vi "cumplimiento.vi"(8 "error in (no error)":errorcluster, 11 "Prueba07 in":refnum<class "Prueba07.lvclass">) -> (0 "error out":errorcluster, 3 "Prueba07 out":refnum<class "Prueba07.lvclass">)   [LabVIEW 2019, in "Prueba07.lvclass"]
uses:
  Prueba07.lvclass
  Prueba07.lvclass/Prueba07.ctl
panel:
  out "cumpimiento":string
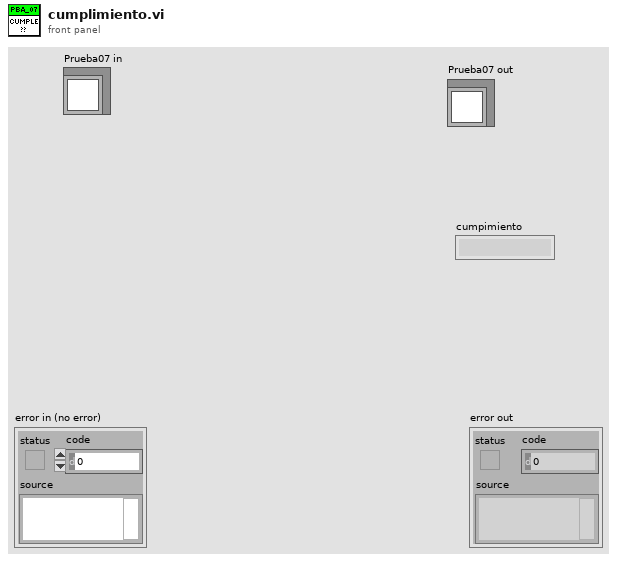
[diagram p1: front panel]
types:
  T1 = cluster{"Medido":dbl, "Error":dbl, "Ref":dbl, "Incert_exp":dbl, "Tol+":dbl, "Tol-":dbl, "fila":i32}
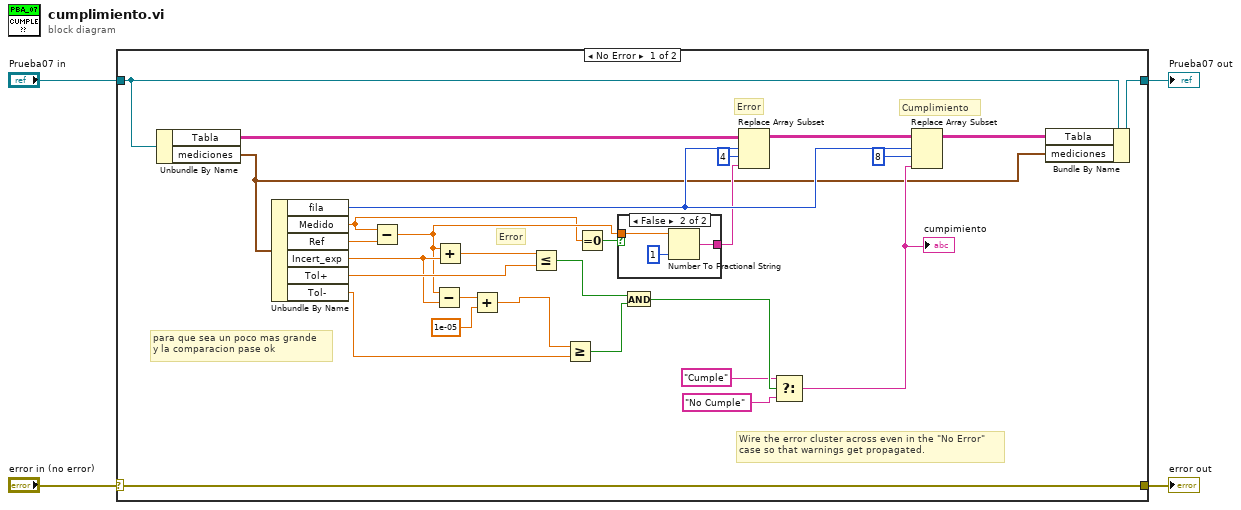
[diagram p0: block diagram]
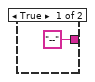
[diagram p2: hidden frame]
diagram:
  n1 = case shown="No Error" "error in (no error)" {
    selector: "error in (no error)" -> [w32 w38]
    tunnel: [w32 w38] -> w3
    tunnel: [w14 w37] -> w2
    tunnel: "Prueba07 in" -> [w12 w37]
    frame No Error {
      # "para que sea un poco mas grande\ny la comparacion pase ok"
      # "Cumplimiento"
      # "Error"
      # "Error"
      # "Wire the error cluster across even in the \"No Error\"\ncase so that warnings get propagated."
      n2 = Unbundle By Name(w12) -> ("Tabla"=w11:string[][], "mediciones"=w10:T1)
      n3 = Unbundle By Name(w10) -> ("fila"=w20:i32, "Medido"=w15:dbl, "Ref"=w26:dbl, "Incert_exp"=w24:dbl, "Tol+"=w25:dbl, "Tol-"=w9:dbl)
      n4 = Subtract(x=w15, y=w26) -> (x-y=w16:dbl)
      n5 = Subtract(x=w16, y=w24) -> (x-y=w8:dbl)
      n6 = Add(x=w16, y=w24) -> (x+y=w31:dbl)
      n7 = Add(x=w8, y=1e-05) -> (x+y=w6:dbl)
      n8 = Less Or Equal?(x=w31, y=w25) -> (x <= y?=w30:bool)
      n9 = Greater Or Equal?(x=w6, y=w9) -> (x >= y?=w5:bool)
      n10 = Equal To 0?(x=w15) -> (x = 0?=w17:bool)
      n11 = case shown="False" w17 {
        tunnel: w16 -> [_ w36]
        tunnel: ["--" w34] -> w18
        frame True {
        }
        frame False {
          n12 = Number To Fractional String(number=w36, precision (6)=i16 1) -> (F-format string=w34:string)  [unwired: 2 in]
        }
      }
      n13 = And(x=w30, y=w5) -> (x .and. y?=w29:bool)
      n14 = Replace Array Subset(array=w11, new element=w18, index (row)=w20, index (col)=4 ("disabled index (col)")) -> (w21:string[][])
      n15 = Select(t="Cumple", s=w29, f="No Cumple") -> (s? t:f=w23:string)
      "cumpimiento" <- w23
      n16 = Replace Array Subset(array=w21, new element=w23, index (row)=w20, index (col)=8 ("index (row)")) -> (w13:string[][])
      n17 = Bundle By Name(cluster=w12, "Tabla"=w13, "mediciones"=w10) -> (w14:refnum<class "Prueba07.lvclass">)
    }
    frame Error {
    }
  }
  "error out" <- w3
  "Prueba07 out" <- w2
